vi "Get Attribute.vi"(7 "Tree ID":string, 8 "Error In":errorcluster, 10 "Attribute Name":string, 11 "Tree Manager":refnum<data-value>) -> (0 "Error Out":errorcluster, 1 "Attribute Value":variant, 2 "Found?":bool, 3 "Tree Manager":refnum<data-value>)   [LabVIEW 2017, in "Tree API.lvlib" / "Tree.lvclass"]
doc: "Get a variant data attribute of the Tree."
uses:
  Tree.lvclass
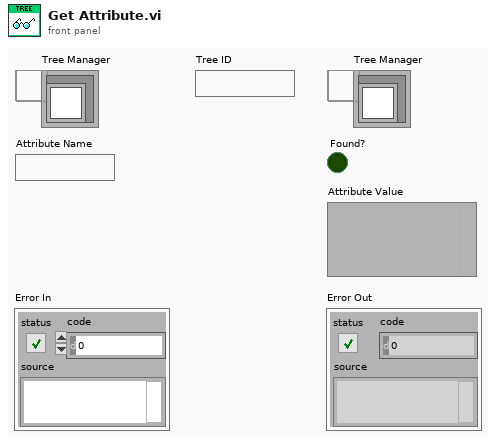
[diagram p1: front panel]
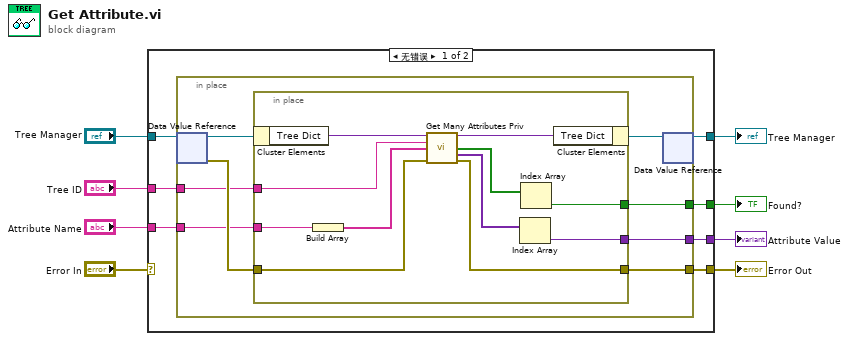
[diagram p0: block diagram]
diagram:
  n1 = case shown="无错误" "Error In" {
    selector: "Error In" -> [_ w35]
    tunnel: "Tree Manager" -> [w15 w36]
    tunnel: [w14 w36] -> w7
    tunnel: [w9 w35] -> w5
    tunnel: "Tree ID" -> [w13 _]
    tunnel: "Attribute Name" -> [w12 _]
    tunnel: [w11 _] -> w2
    tunnel: [w10 _] -> w1
    frame No Error {
      n2 = in-place {
        in-place-border: w13 -> [w20]
        in-place-border: w12 -> [w19]
        in-place-border: [w18] -> w11
        in-place-border: [w17] -> w10
        in-place-border: [w16] -> w9
        n3 = in-place-dvr #1(w15) -> (w23:refnum<class "Tree.lvclass">, w21:errorcluster)
        n4 = in-place {
          in-place-border: w21 -> [w25]
          in-place-border: w20 -> [w27]
          in-place-border: w19 -> [w28]
          in-place-border: [w30] -> w18
          in-place-border: [w29] -> w17
          in-place-border: [w24] -> w16
          n5 = in-place-cluster #2(w23) -> ("Tree Dict"=w34:variant)
          n6 = Build Array(w28) -> (w26:string[])
          n7 = call "Get Many Attributes Priv.vi"("Tree Dictionary In"=w34, "Unique ID"=w27, "Attribute Names"=w26, "error in"=w25) -> ("Tree Dictionary Out"=w33:variant, "Found?"=w32:bool[], "Attribute Values"=w31:variant[], "error out"=w24:errorcluster)  [unwired: 6 in, 2 out]
          n8 = Index Array(array=w31) -> (element=w29:variant)  [unwired: 1 in]
          n9 = Index Array(array=w32) -> (element=w30:bool)  [unwired: 1 in]
          n10 = in-place-cluster #2("Tree Dict"=w33) -> (w22:refnum<class "Tree.lvclass">)
        }
        n11 = in-place-dvr #1(w22) -> (w14:refnum<data-value>)  [unwired: 1 out]
      }
    }
    frame Error {
    }
  }
  "Tree Manager" <- w7
  "Error Out" <- w5
  "Found?" <- w2
  "Attribute Value" <- w1
